vi "XTAL Cal.vi"(8 "error in (no error)":errorcluster, 11 "XtalCalConfig":T1) -> (0 "error out":errorcluster, 3 "return type":i32)   [LabVIEW 2015, in "QCA_DUT_Func.lvlib"]
doc: "DLL_QMSL_AEROFLEX void _stdcall XTALCal(int channel, int txChain0, int iXtalTargetPPM, unsigned int iXtalTolerancePPM, int numMeasAvg );"
uses:
  QCA_DUT_Func.lvlib
  QCA_DUT_Func.dll
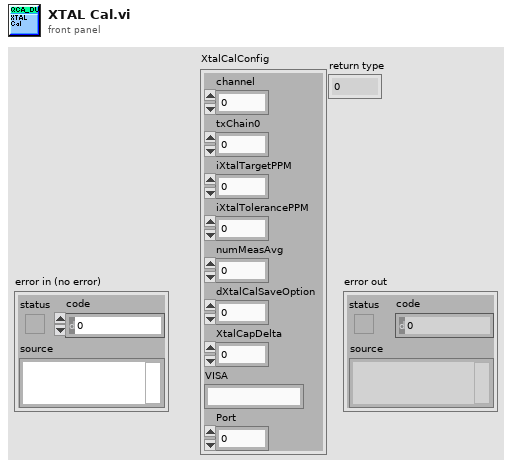
[diagram p1: front panel]
types:
  T1 = cluster{"channel":i32, "txChain0":i32, "iXtalTargetPPM":i32, "iXtalTolerancePPM":u32, "numMeasAvg":u32, "dXtalCalSaveOption":u32, "XtalCapDelta":i32, "VISA":string, "Port":i32}
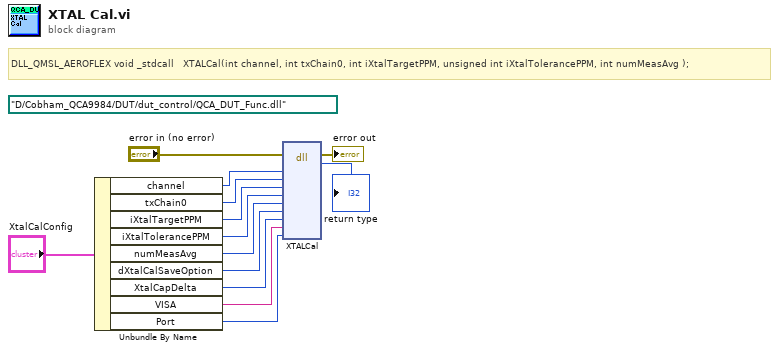
[diagram p0: block diagram]
diagram:
  (unwired) path "D:/Cobham_QCA9984/DUT/dut_control/QCA_DUT_Func.dll" ("path in")
  # "DLL_QMSL_AEROFLEX void _stdcall   XTALCal(int channel, int txChain0, int iXtalTargetPPM, unsigned int iXtalTolerancePPM, int numMeasAvg );"
  n1 = Unbundle By Name("XtalCalConfig") -> ("channel"=w10:i32, "txChain0"=w9:i32, "iXtalTargetPPM"=w8:i32, "iXtalTolerancePPM"=w7:u32, "numMeasAvg"=w6:u32, "dXtalCalSaveOption"=w5:u32, "XtalCapDelta"=w4:i32, "VISA"=w3:string, "Port"=w2:i32)
  n2 = dll-call lib="D:/4-Up-WLAN-Test-System/DUT Control/DUT/dut_control/QCA_DUT_Func.dll" fn="XTALCal"(error in="error in (no error)", "channel"=w10, "txChain0"=w9, "iXtalTargetPPM"=w8, "iXtalTolerancePPM"=w7, "dXtalCalSaveOption"=w6, "XtalCapDelta"=w5, "numMeasAvg"=w4, "VISA"=w3, "Port"=w2) -> (error out=→"error out":errorcluster, "return type"=→"return type":i32)  [unwired: 11 in, 1 out]
